vi "Fiducial Parameters Finder From File.vi"() -> ()   [LabVIEW 2011]
uses:
  Shared Components/gVision API/gVision/gVision.lvlib
panel:
  in  "Fiducial Parameters":T1
  out "error out":errorcluster
  out "Preview":T2(plugin-control)
  in  "Display Steps":bool
  out "Result":T2(plugin-control)
  out "ficucial coordinates":cluster{"x":dbl, "y":dbl}[](array[cluster])
  in  "Input Image Path":path=path "C:/Users/husker/Desktop/sample_potting_images/good_ref_potting1.jpg"
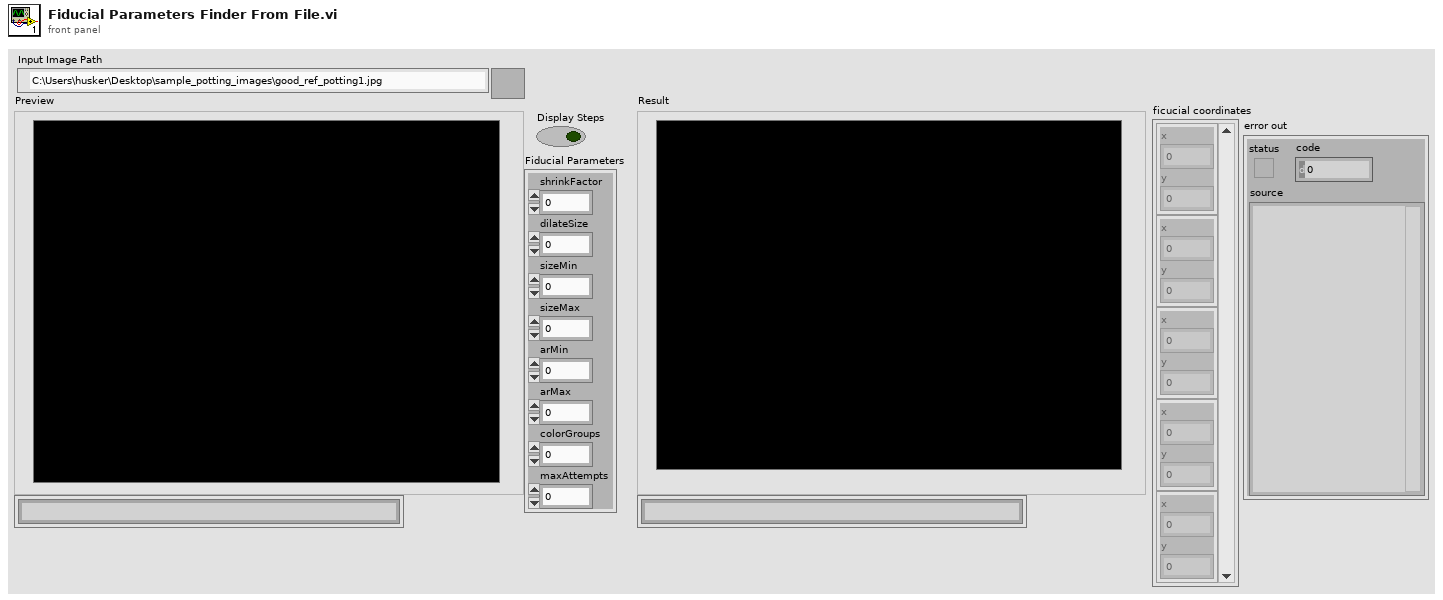
[diagram p1: front panel]
types:
  T1 = cluster{"shrinkFactor":sgl, "dilateSize":i32, "sizeMin":sgl, "sizeMax":sgl, "arMin":sgl, "arMax":sgl, "colorGroups":i32, "maxAttempts":i32}
  T2 = typedef "IMAQ Image.ctl" = refnum<image>
  T3 = cluster{"Left":i32, "Top":i32, "Right":i32, "Bottom":i32}
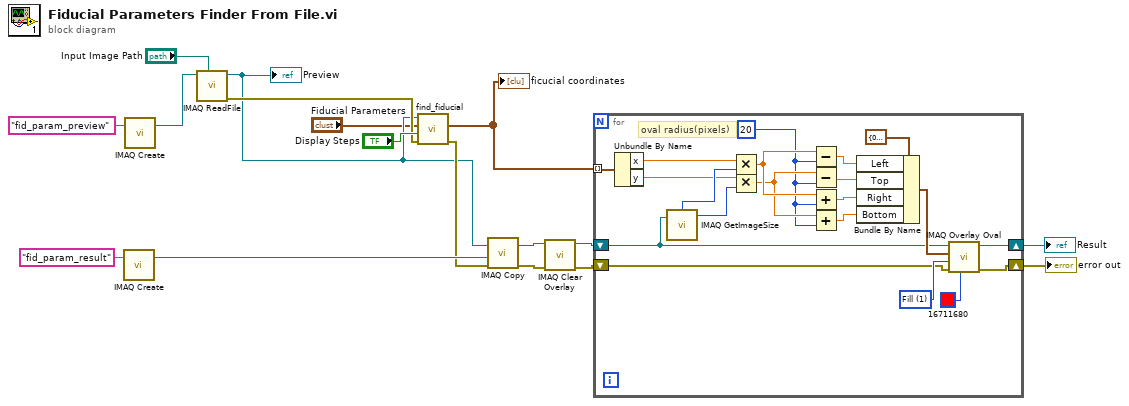
[diagram p0: block diagram]
diagram:
  n1 = call "IMAQ Create"("Image Name"="fid_param_result") -> ("New Image"=w15:T2)  [unwired: 4 in, 1 out]
  n2 = call "IMAQ Create"("Image Name"="fid_param_preview") -> ("New Image"=w5:T2)  [unwired: 4 in, 1 out]
  n3 = call "IMAQ ReadFile"("File Path"="Input Image Path", "Image"=w5) -> ("error out"=w4:errorcluster, "Image Out"=w3:T2)  [unwired: 5 in, 3 out]
  "Preview" <- w3
  n4 = call "find_fiducial.vi"("error in"=w4, "interactive"="Display Steps", "Fiducial Parameters"="Fiducial Parameters", "Image"=w3) -> ("error out"=w11:errorcluster, "coords"=w12:cluster{"x":dbl, "y":dbl}[])  [unwired: 6 in]
  "ficucial coordinates" <- w12
  n5 = call "IMAQ Copy"("error in (no error)"=w11, "Image Dst"=w15, "Image Src"=w3) -> ("error out"=w9:errorcluster, "Image Dst Out"=w10:T2)  [unwired: 3 in]
  n6 = call "IMAQ Clear Overlay"("error in (no error)"=w9, "Image"=w10) -> ("error out"=w7:errorcluster, "Image Out"=w8:T2)  [unwired: 8 in]
  n7 = for {
    tunnel: w12 -> [w33] mode=indexing
    shift-right: [w37] -> w14
    shift-left: w8 -> [w29]
    shift-right: [w31] -> w2
    shift-left: w7 -> [w30]
    w18 = 20
    w32 = u32 1 items=["Frame", "Fill"] ("Drawing Mode (Frame)")
    # "oval radius(pixels)"
    n8 = Unbundle By Name(w33) -> ("x"=w27:dbl, "y"=w25:dbl)
    n9 = call "IMAQ GetImageSize"("Image"=w29) -> ("Y Resolution"=w26:i32, "X Resolution"=w28:i32)  [unwired: 3 in, 1 out]
    n10 = Multiply(x=w27, y=w28) -> (x*y=w20:dbl)
    n11 = Multiply(x=w25, y=w26) -> (x*y=w19:dbl)
    n12 = Subtract(x=w20, y=w18) -> (x-y=w24:dbl)
    n13 = Subtract(x=w19, y=w18) -> (x-y=w23:dbl)
    n14 = Add(x=w20, y=w18) -> (x+y=w22:dbl)
    n15 = Add(x=w19, y=w18) -> (x+y=w21:dbl)
    n16 = Bundle By Name(cluster=T3 {"Left"=0, "Top"=0, "Right"=0, "Bottom"=0} ("Bounding Rectangle"), "Left"=w24, "Top"=w23, "Right"=w22, "Bottom"=w21) -> (w34:T3)
    n17 = call "IMAQ Overlay Oval"("Color"=u32 16711680, "error in (no error)"=w30, "Drawing Mode (Frame)"=w32, "Bounding Rectangle"=w34, "Image"=w29) -> ("error out"=w31:errorcluster, "Image Out"=w37:T2)  [unwired: 5 in]
  }
  "error out" <- w2
  "Result" <- w14
